vi "Auto 1.vi"(8 "Error In":errorcluster) -> (0 "Error Out":errorcluster)   [LabVIEW 2014]
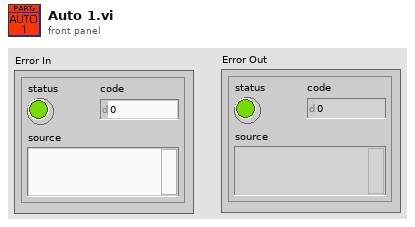
[diagram p1: front panel]
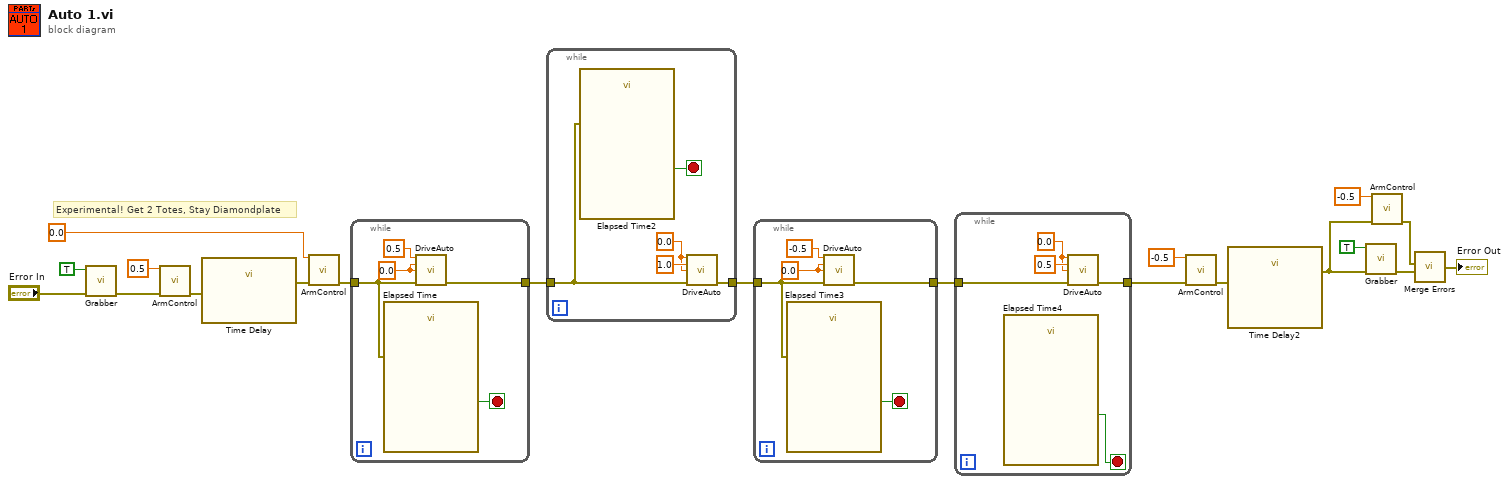
[diagram p0: block diagram]
diagram:
  # "Experimental! Get 2 Totes, Stay Diamondplate"
  n1 = call "Grabber.vi"("Error In"="Error In", "Grabber Open/Close"=TRUE) -> ("Error Out"=w11:errorcluster)  [unwired: 9 in]
  n2 = call "ArmControl.vi"("Arm Value"=0.5, "Error In"=w11) -> ("Error Out"=w12:errorcluster)  [unwired: 13 in]
  n3 = call "Time Delay"("error in (no error)"=w12) -> ("error out"=w13:errorcluster)  [unwired: 10 in]
  n4 = call "ArmControl.vi"("Arm Value"=0.0, "Error In"=w13) -> ("Error Out"=w15:errorcluster)  [unwired: 13 in]
  n5 = while {
    tunnel: w15 -> [w22]
    tunnel: [w21] -> w14
    stop <- w23 stop-if-true
    w24 = 0.0 ("Arm Value")
    n6 = call "Elapsed Time"("error in (no error)"=w22) -> ("Time has Elapsed"=w23:bool)  [unwired: 11 in, 7 out]
    n7 = call "DriveAuto.vi"("X In"=0.5, "Y In"=w24, "R In"=w24, "Error In"=w22) -> ("Error Out"=w21:errorcluster)  [unwired: 11 in]
  }
  n8 = while {
    tunnel: w14 -> [w28]
    tunnel: [w27] -> w16
    stop <- w29 stop-if-true
    w26 = 0.0 ("X In")
    n9 = call "Elapsed Time2"("error in (no error)"=w28) -> ("Time has Elapsed"=w29:bool)  [unwired: 11 in, 7 out]
    n10 = call "DriveAuto.vi"("X In"=w26, "Y In"=1.0 ("Arm Value"), "R In"=w26, "Error In"=w28) -> ("Error Out"=w27:errorcluster)  [unwired: 11 in]
  }
  n11 = while {
    tunnel: w16 -> [w32]
    tunnel: [w31] -> w17
    stop <- w33 stop-if-true
    w34 = 0.0 ("Arm Value")
    n12 = call "Elapsed Time3"("error in (no error)"=w32) -> ("Time has Elapsed"=w33:bool)  [unwired: 11 in, 7 out]
    n13 = call "DriveAuto.vi"("X In"=-0.5, "Y In"=w34, "R In"=w34, "Error In"=w32) -> ("Error Out"=w31:errorcluster)  [unwired: 11 in]
  }
  n14 = while {
    tunnel: w17 -> [w39]
    tunnel: [w38] -> w19
    stop <- w36 stop-if-true
    w37 = 0.0 ("X In")
    n15 = call "Elapsed Time4"() -> ("Time has Elapsed"=w36:bool)  [unwired: 12 in, 7 out]
    n16 = call "DriveAuto.vi"("X In"=w37, "Y In"=0.5 ("Arm Value"), "R In"=w37, "Error In"=w39) -> ("Error Out"=w38:errorcluster)  [unwired: 11 in]
  }
  n17 = call "ArmControl.vi"("Arm Value"=-0.5, "Error In"=w19) -> ("Error Out"=w18:errorcluster)  [unwired: 13 in]
  n18 = call "Time Delay2"("error in (no error)"=w18) -> ("error out"=w20:errorcluster)  [unwired: 10 in]
  n19 = call "Grabber.vi"("Error In"=w20, "Grabber Open/Close"=TRUE) -> ("Error Out"=w2:errorcluster)  [unwired: 9 in]
  n20 = call "ArmControl.vi"("Arm Value"=-0.5, "Error In"=w20) -> ("Error Out"=w3:errorcluster)  [unwired: 13 in]
  n21 = call "Merge Errors.vi"("error in 2"=w2, "error in"=w3) -> ("error out"=→"Error Out":errorcluster)  [unwired: 2 in]
